vi "Title_Move.vi"(2 "error in (no error)":errorcluster caption="错误输入（无错误）", 3 "本VI":refnum<vi>) -> (0 "error out":errorcluster caption="错误输出")   [LabVIEW 2012]
uses:
  <vilib>/Utility/inputDevices.llb/mouseAcquire.vi
  <vilib>/Utility/inputDevices.llb/closeMouse.vi
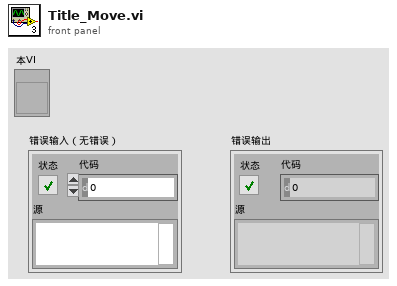
[diagram p1: front panel]
types:
  T1 = cluster{"Horizontal":i32, "Vertical":i32, "Scrolling":i32}
  T2 = typedef "LVRectTypeDef.ctl" = cluster{"Left":i16, "Top":i16, "Right":i16, "Bottom":i16}
  T3 = cluster{"Horizontal":i32, "Vertical":i32, "Horizontal":i32, "Vertical":i32}
  T4 = cluster{"button 1":bool, "button 2":bool, "button 3":bool, "button 4":bool}
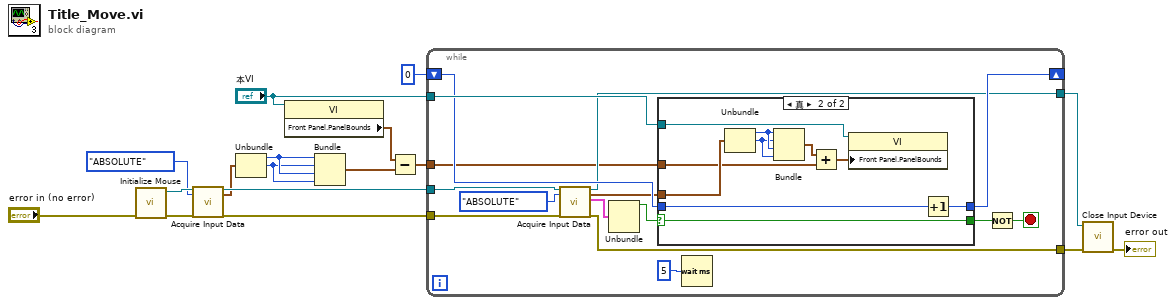
[diagram p0: block diagram]
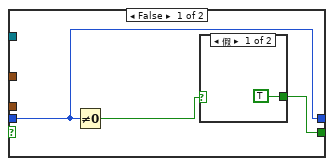
[diagram p2: hidden frame]
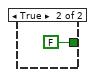
[diagram p3: hidden frame]
diagram:
  n1 = call <vilib>:"Initialize Mouse.vi"("error in (no error)"="error in (no error)") -> ("error out"=w10:errorcluster, "device ID"=w17:refnum<k1>)  [unwired: 9 in]
  n2 = call-poly <vilib>:"Acquire Input Data.vi"("device ID"=w17, "key mode"=enum16{"RELATIVE", "ABSOLUTE"}."ABSOLUTE", "error in (no error)"=w10) -> ("device ID"=w11:refnum<k1>, "axis info"=w8:T1, "error out"=w9:errorcluster)  [unwired: 13 in, 1 out]
  n3 = Unbundle(w8) -> ("Horizontal"=w6:i32, "Vertical"=w5:i32)  [unwired: 1 out]
  n4 = property class="VI"(reference="本VI") -> ("Front Panel.PanelBounds"=w4:T2)  [unwired: 1 in, 2 out]
  n5 = Bundle("Horizontal"=w6, "Vertical"=w5, "Horizontal"=w6, "Vertical"=w5) -> (w3:T3)  [unwired: 1 in]
  n6 = Subtract(x=w4, y=w3) -> (x-y=w2:cluster{i32, i32, i32, i32})
  n7 = while {
    tunnel: w11 -> [w31]
    tunnel: w9 -> [w30]
    tunnel: [w20] -> w16
    tunnel: [w29] -> w15
    tunnel: "本VI" -> [w25]
    shift-right: [w21] -> _
    shift-left: u32 0 ("等待时间（毫秒）") -> [w22]
    tunnel: w2 -> [w18]
    stop <- w23 stop-if-true
    n8 = call-poly <vilib>:"Acquire Input Data.vi"("device ID"=w31, "key mode"=enum16{"RELATIVE", "ABSOLUTE"}."ABSOLUTE", "error in (no error)"=w30) -> ("device ID"=w20:refnum<k1>, "axis info"=w19:T1, "button info"=w28:T4, "error out"=w29:errorcluster)  [unwired: 13 in]
    n9 = Unbundle(w28) -> ("button 1"=w27:bool)  [unwired: 3 out]
    n10 = case shown="真" w27 {
      selector: w27 -> [_ w47]
      tunnel: w25 -> [_ w44]
      tunnel: [w35 w47] -> w24
      tunnel: w22 -> [w33 w46]
      tunnel: [w33 w45] -> w21
      tunnel: w19 -> [_ w41]
      tunnel: w18 -> [_ w39]
      frame False {
        n11 = Not Equal To 0?(x=w33) -> (x != 0?=w34:bool)
        n12 = case shown="假" w34 {
          tunnel: [TRUE FALSE] -> w35
          frame False {
          }
          frame True {
          }
        }
      }
      frame True {
        n13 = Unbundle(w41) -> ("Horizontal"=w43:i32, "Vertical"=w42:i32)  [unwired: 1 out]
        n14 = Bundle("Horizontal"=w43, "Vertical"=w42, "Horizontal"=w43, "Vertical"=w42) -> (w40:T3)  [unwired: 1 in]
        n15 = Add(x=w40, y=w39) -> (x+y=w38:cluster{i32, i32, i32, i32})
        n16 = property class="VI"(reference=w44, "Front Panel.PanelBounds"=w38) -> ()  [unwired: 1 in, 2 out]
        n17 = Increment(x=w46) -> (x+1=w45:u32)
      }
    }
    n18 = Wait (ms)(milliseconds to wait=u32 5 ("等待时间（毫秒）")) -> ()  [unwired: 1 out]
    n19 = Not(x=w24) -> (.not. x?=w23:bool)
  }
  n20 = call-poly <vilib>:"Close Input Device.vi"("error in (no error)"=w15, "device ID"=w16) -> ("error out"=→"error out":errorcluster)  [unwired: 8 in]
